vi "ORS_Insight_Reduce_Data_with_Valid-Vector.vi"(9 "Valid Vector":i16[](array[numeric]), 10 "DVV shift":i16, 11 "Raw Data":i16[](array[numeric])) -> (3 "Valid Data":i16[](array[numeric]))   [LabVIEW 2021]
doc: "Insight Photonic Solutions\n\nver 1.0 - original release\n\nThis VI inputs raw data from an acquisition with the laser and outputs Valid Data, that is cleaned of the hold points in the sweep (sporadically during a sweep). The valid data are located at indices given by the \"Valid Vector\".\n\nHow to use this VI:\n1. After a sweep calibration is performed, request the Indices of the Invalid Data Points from the laser. These indices will be correct until the next time a sweep calibration is performed.\n\n2. Construct the Valid Vector, using \"Insight_Create_Valid_Vector.vi\", before beginning a data acquisition sequence. You only need to do this once, right after the sweep calibration. This saves time in data processing and allows the data to flow quickly from the Data Acquisition card to your image processing code.\n\n3. For each data acquisition, send the Raw Data from the Data Acquisition card to this vi \"Insight_Reduce_Data_with_Valid-Vector.vi\".\n\n4. Send the \"Valid Data\" to your image processing software."
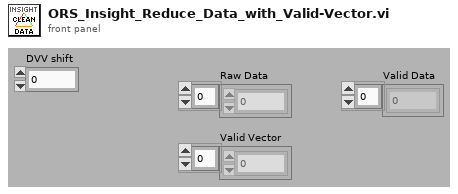
[diagram p1: front panel]
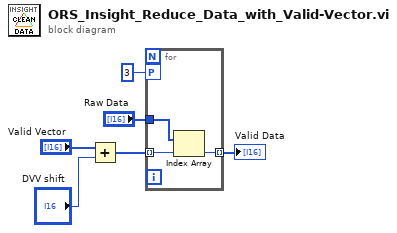
[diagram p0: block diagram]
diagram:
  n1 = Add(x="Valid Vector", y="DVV shift") -> (x+y=w1:i16[])
  n2 = for {
    tunnel: "Raw Data" -> [w9]
    tunnel: w1 -> [w8] mode=indexing
    tunnel: [w7] -> w4 mode=indexing
    workers-P: 3 -> [_]
    n3 = Index Array(array=w9, index=w8) -> (element=w7:i16)
  }
  "Valid Data" <- w4
